vi "map_trap_switch_laser.vi"() -> ()   [LabVIEW 2015]
panel:
  out "Mapping file":string
  in  "Done ?":bool
  in  "KILL":bool
  in  "PAUSE":bool
  in  "RESUME":bool
  in  "QUIT":bool
  in  "up done":bool
  in  "z up":bool
  in  "Done":bool
  in  "z piastra":bool
  in  "y piastra":bool
  in  "x piastra":bool
  in  "goto x pos":bool
  in  "Panello o piastre?":bool
  in  "End":bool
  in  "zero z - end":bool
  in  "zero x - end":bool
  in  "zero y - end":bool
  in  "goto z pos":bool
  in  "positioning done":bool
  out "output":string
  out "command":string
  in  "zero done":bool
  in  "zero z":bool
  in  "zero x":bool
  in  "zero y":bool
  # "Comandi di emergenza"
  # "Mappatura a trapezio \nper il pannello e le piastre"
  # "In alto: TRUE ---> Panello"
  # "In basso: FALSE ---> Piastre"
  # "Posiziono in zero"
  # "Vado sulla piastra \ne azzero"
  # "Alzo il laser"
  # "Vado in posizione"
  # "Ritorno a zero"
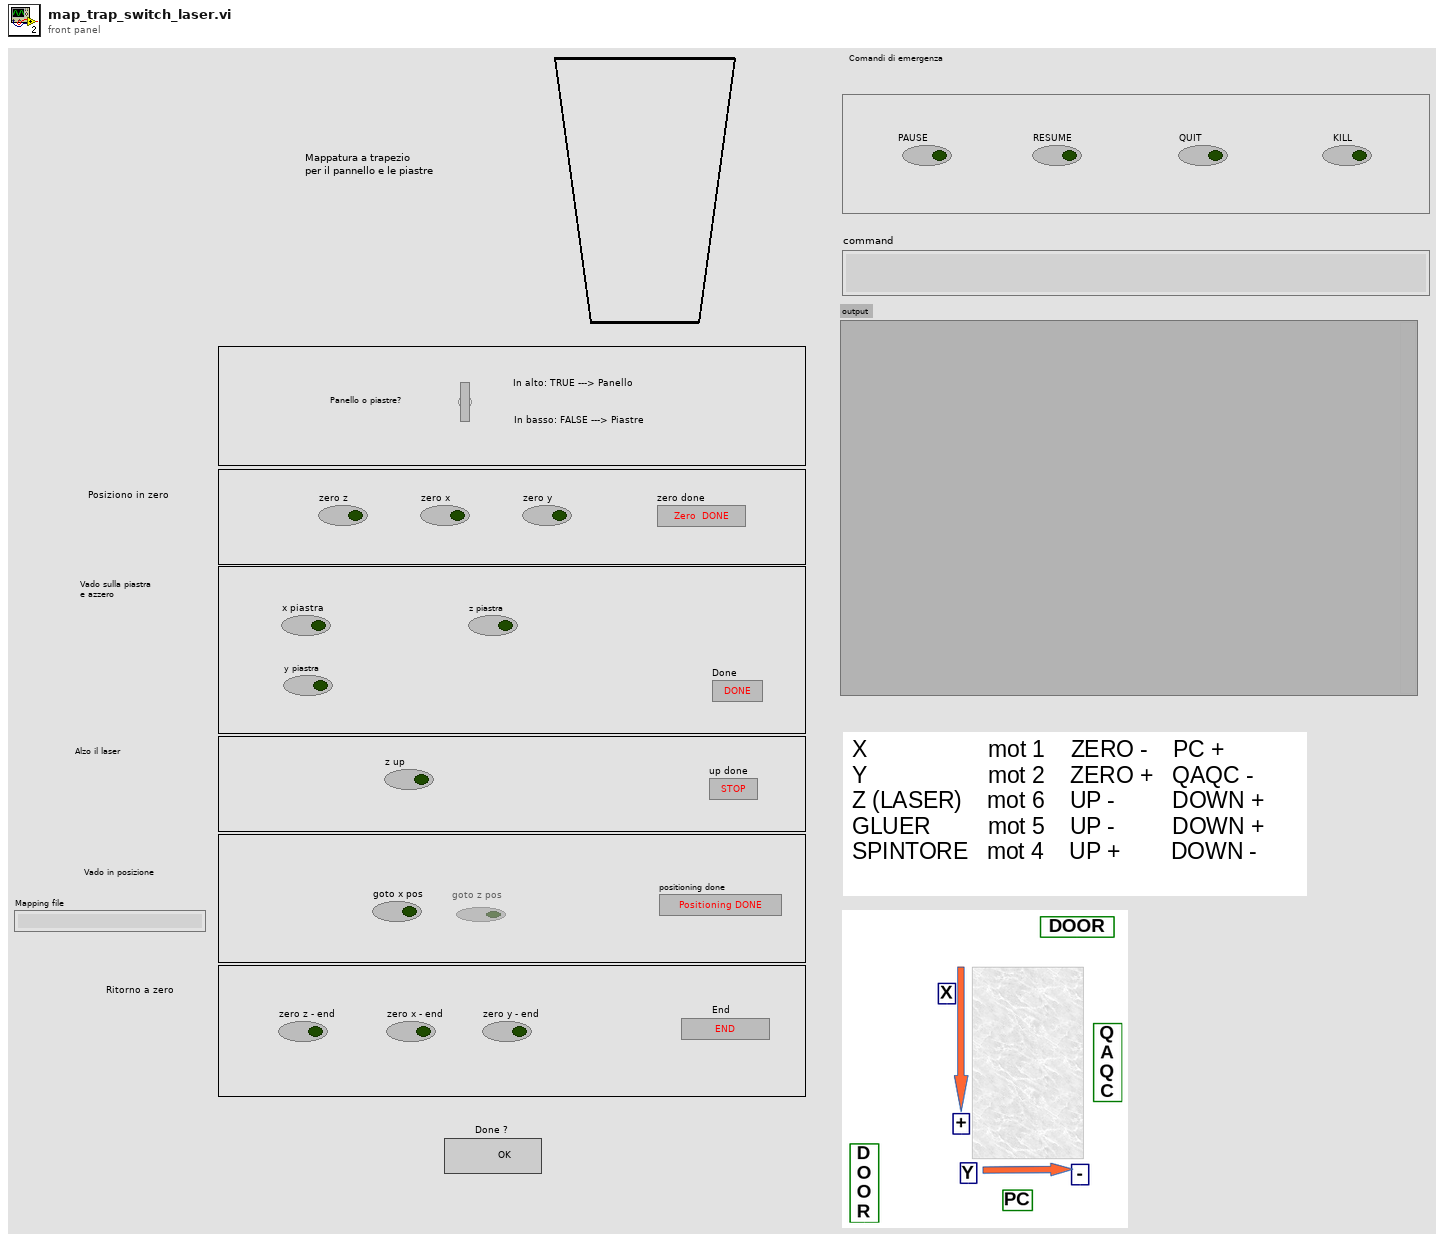
[diagram p1: front panel]
types:
  T1 = enum8{"Enabled", "Disabled", "Disabled and Grayed Out"}
  T2 = enum16{"open", "replace", "create", "open or create", "replace or create", "replace or create with confirmation"}
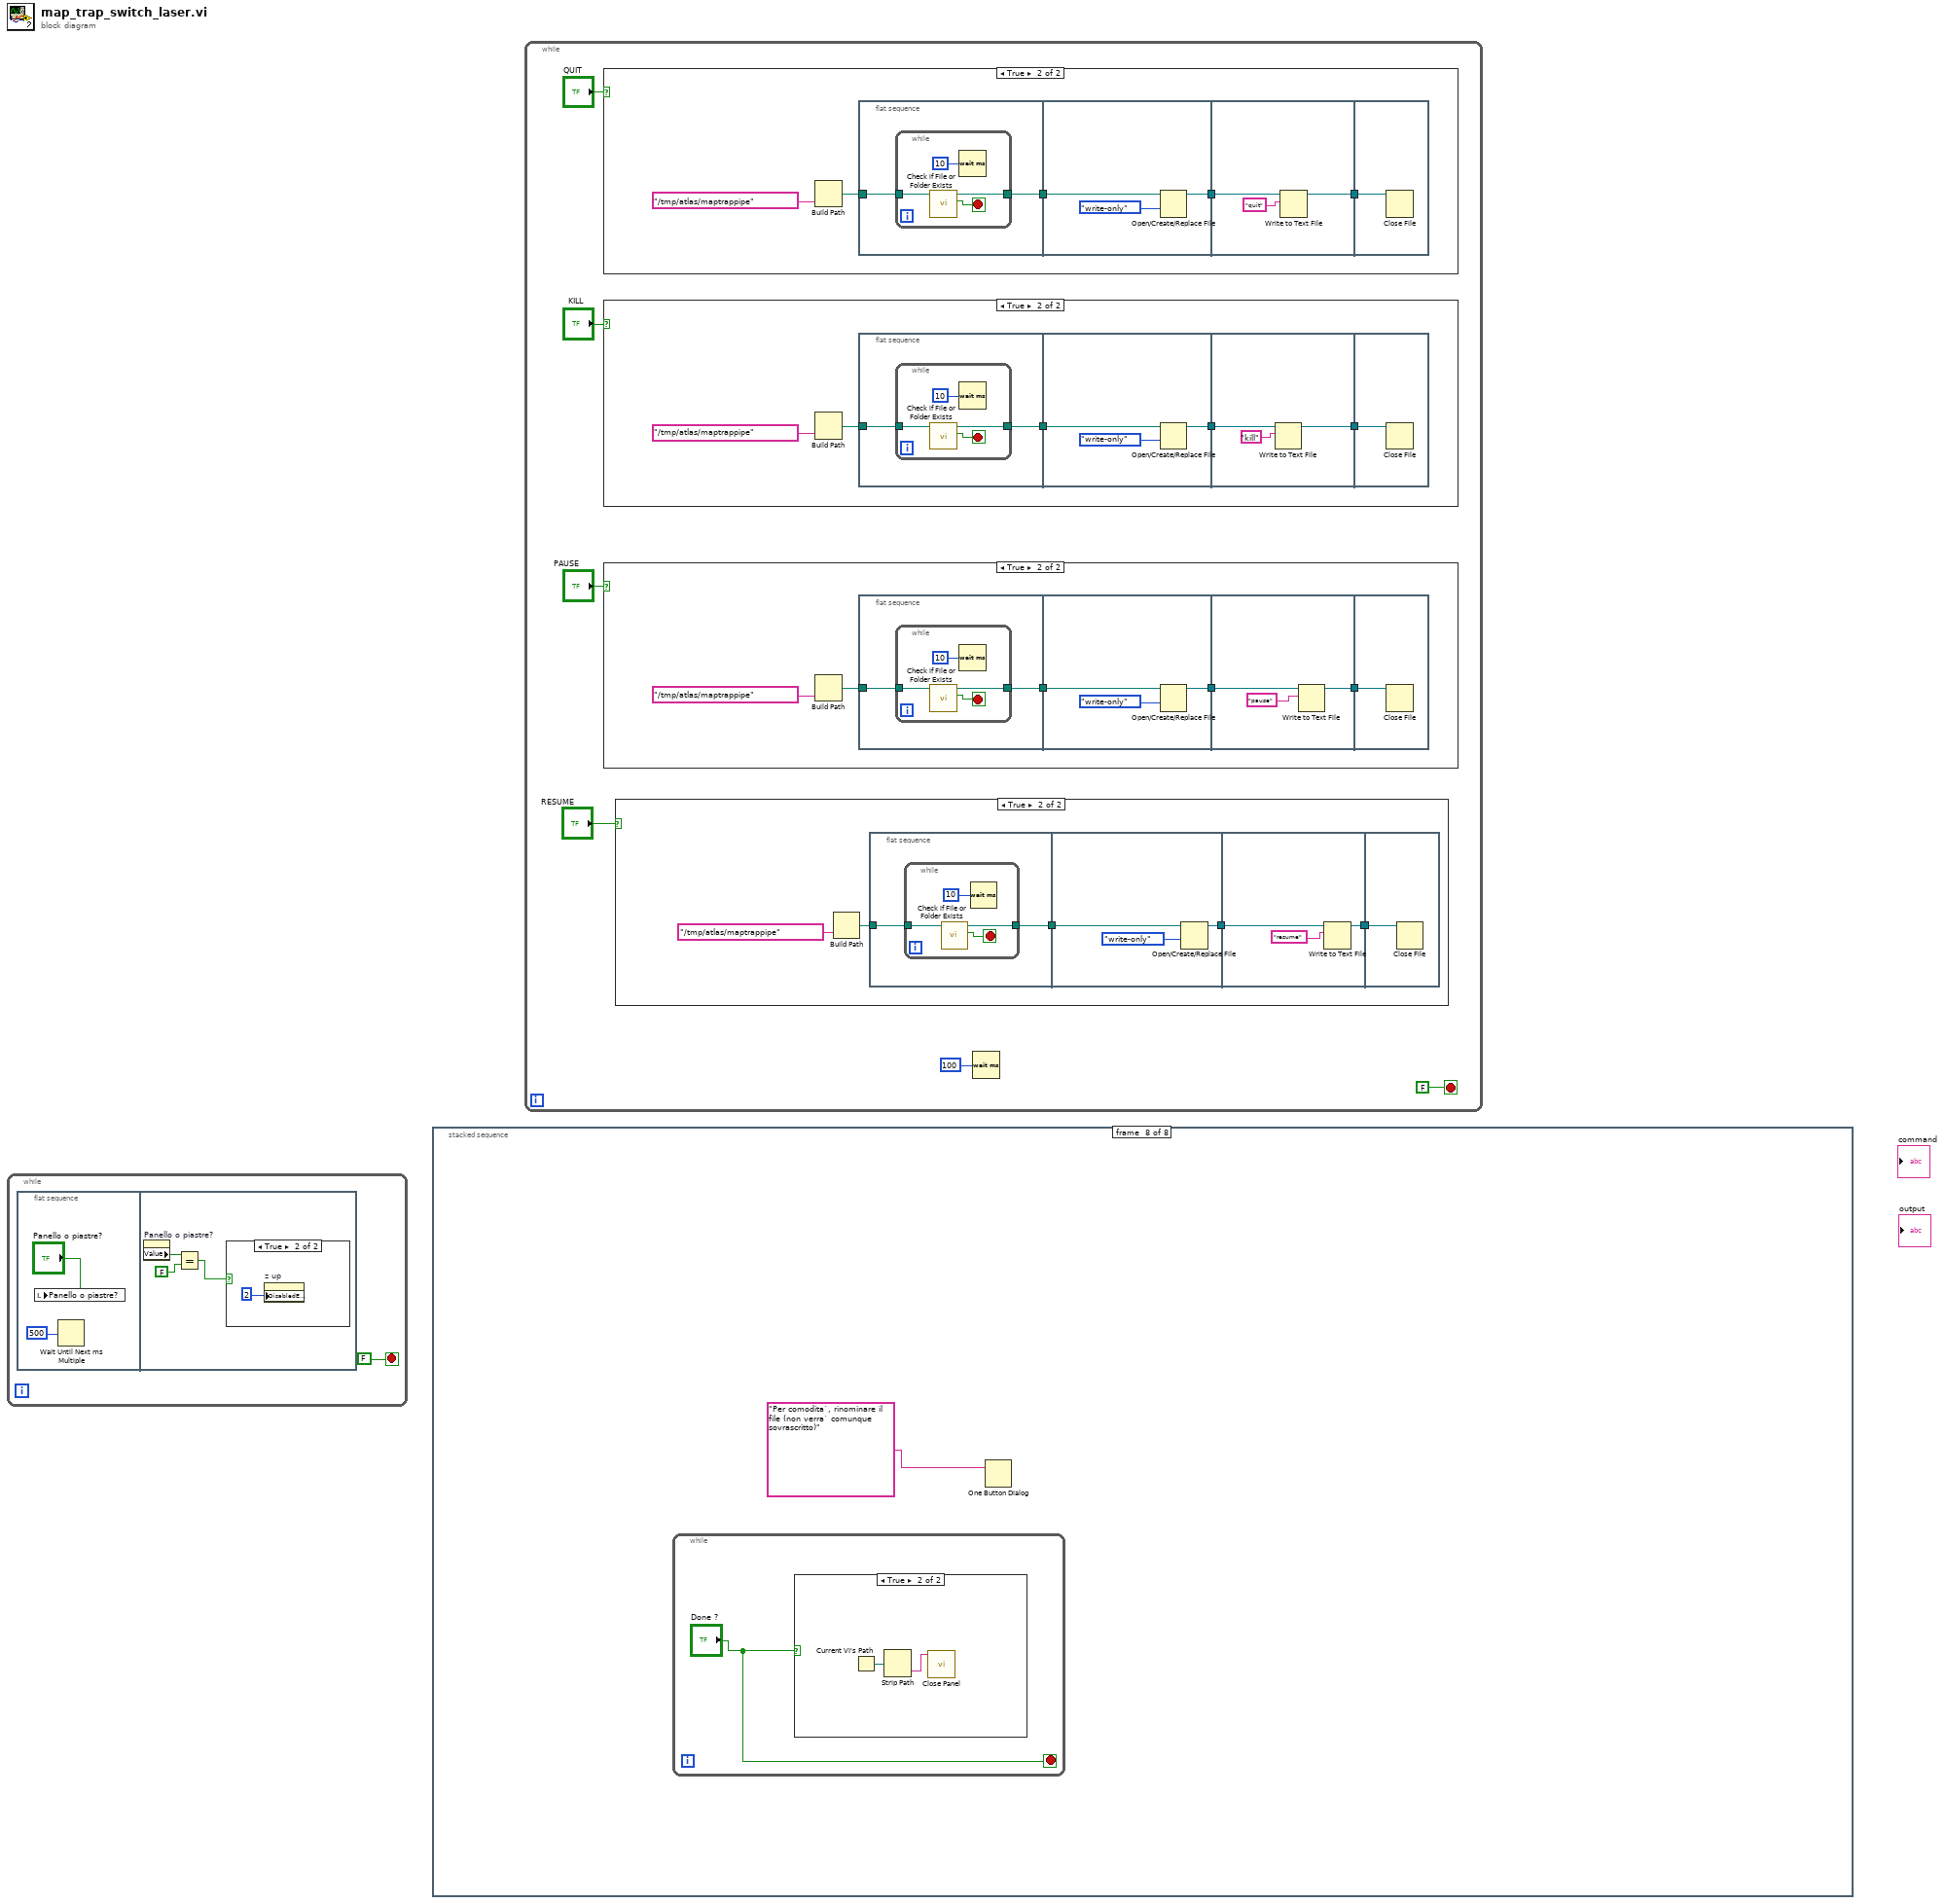
[diagram p0: block diagram]
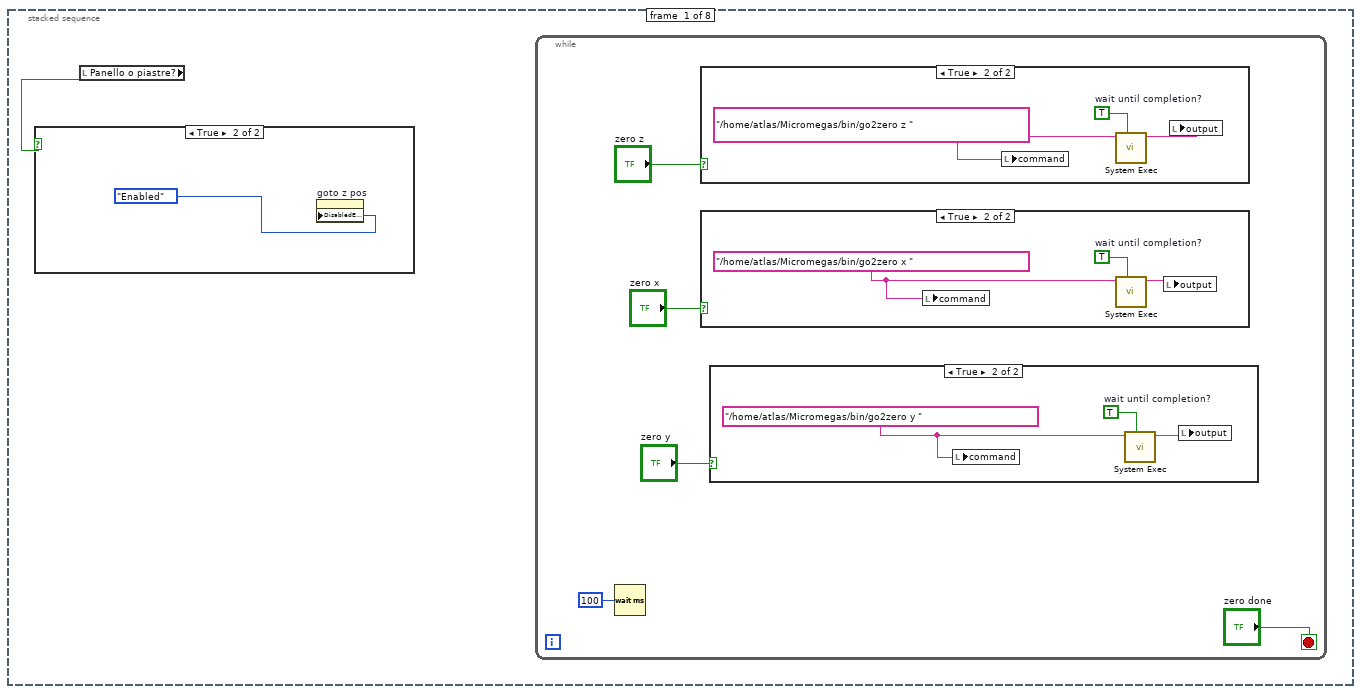
[diagram p7: hidden frame]
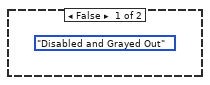
[diagram p8: hidden frame]
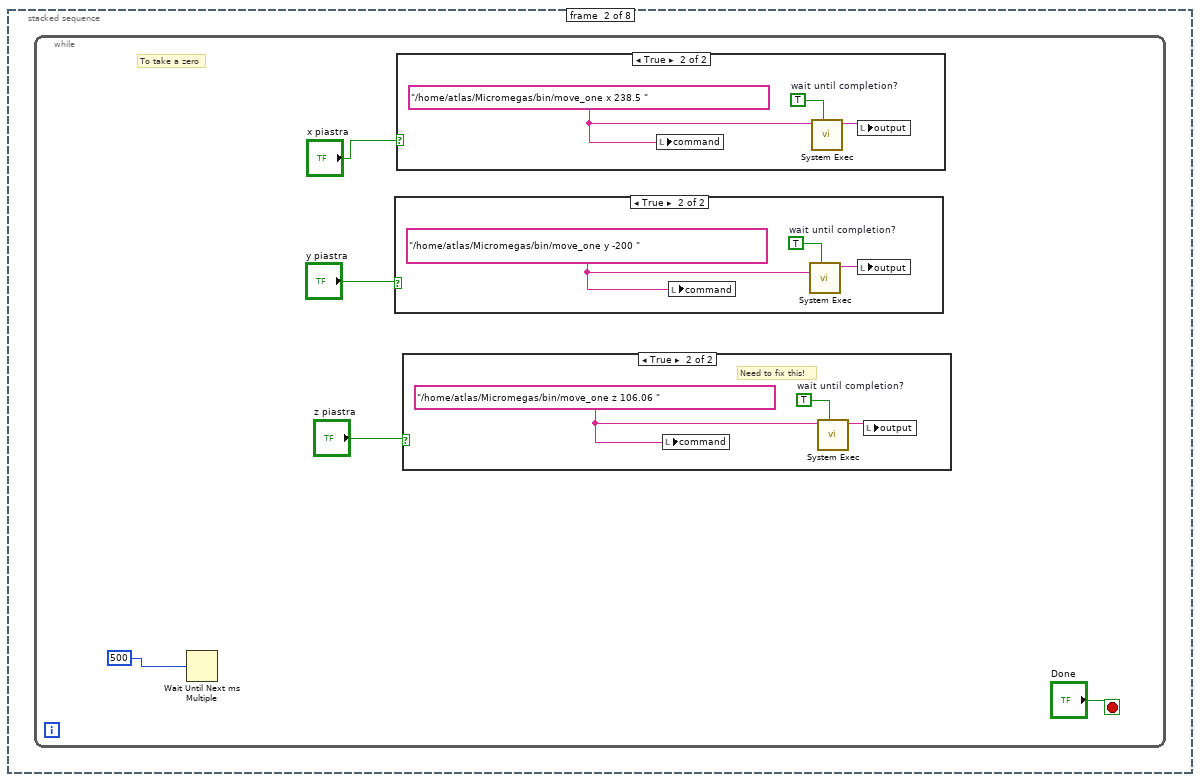
[diagram p12: hidden frame]
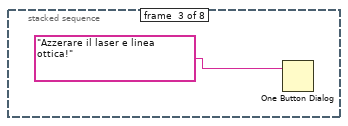
[diagram p16: hidden frame]
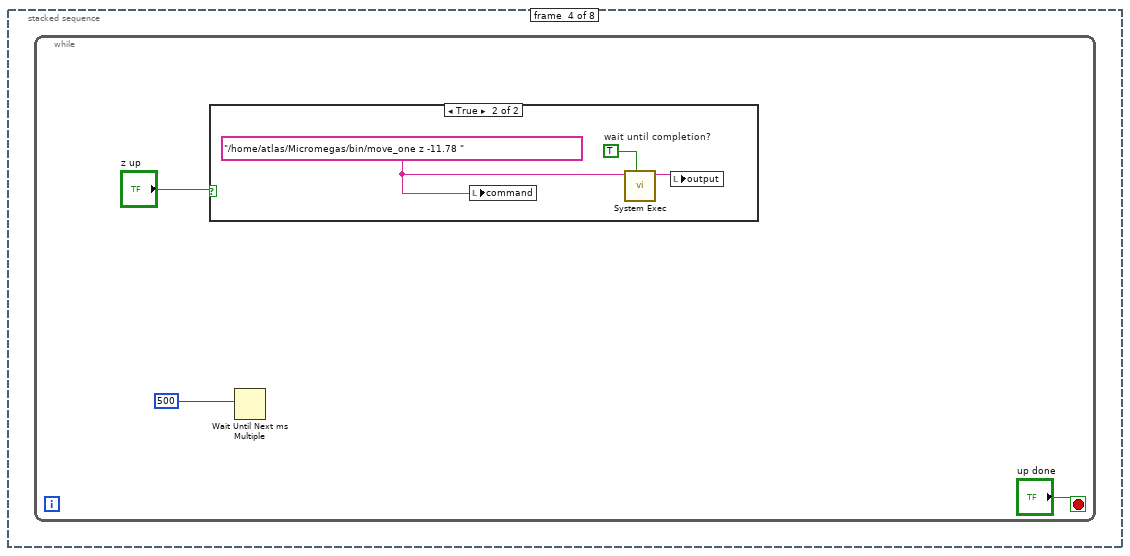
[diagram p17: hidden frame]
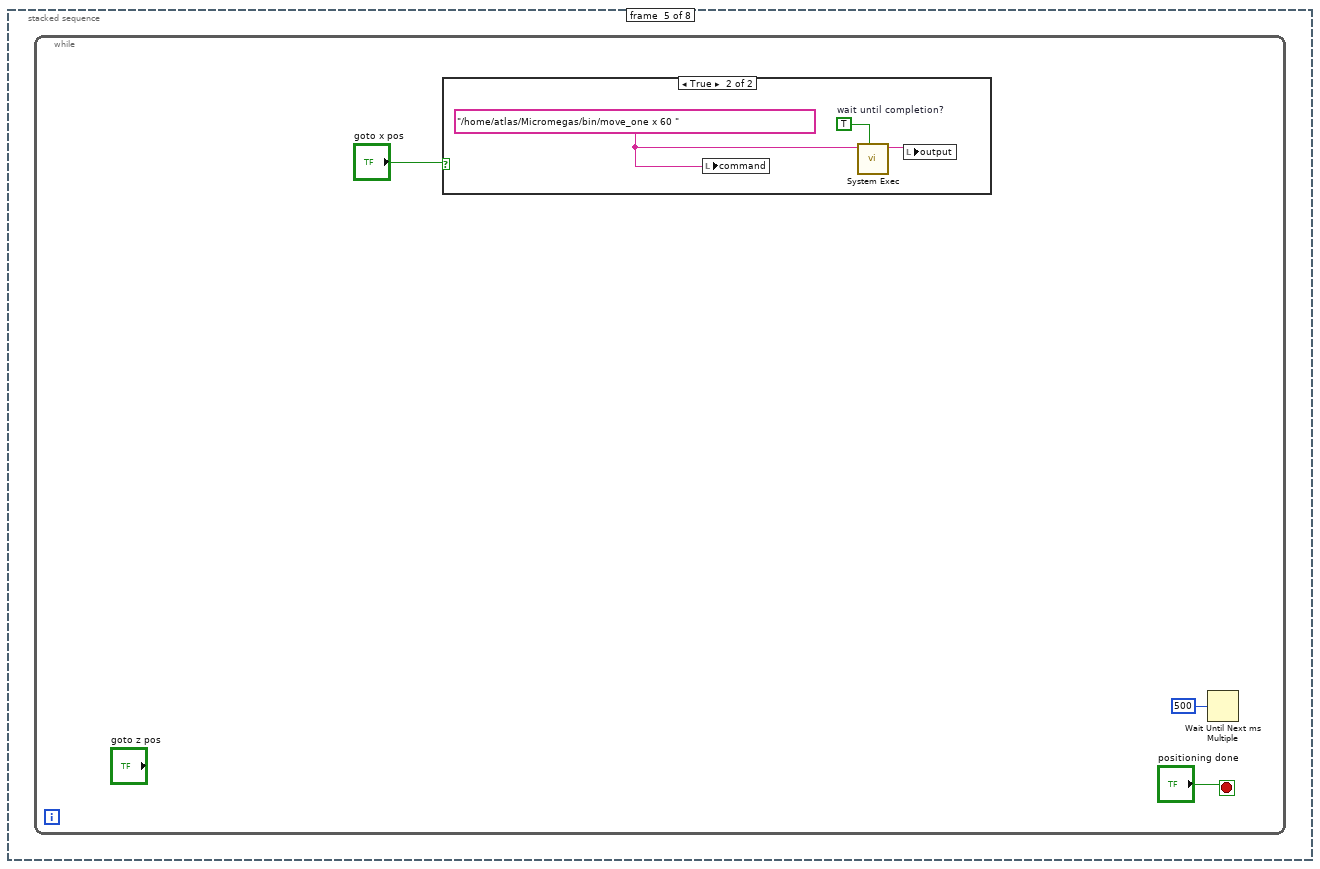
[diagram p19: hidden frame]
diagram:
  n1 = while {
    stop <- FALSE stop-if-true
    n2 = flat-sequence {
      frame #0 {
        n3 = local write "Panello o piastre?"("Panello o piastre?") -> ()
        n4 = Wait Until Next ms Multiple(millisecond multiple=u32 500) -> ()  [unwired: 1 out]
      }
      frame #1 {
        n5 = property on="Panello o piastre?" class="Bool (strict)"() -> ("Value"=w6:bool)  [unwired: 2 in, 2 out]
        n6 = Equal?(x=w6, y=FALSE) -> (x = y?=w4:bool)
        n7 = case shown="True" w4 {
          frame False {
          }
          frame True {
            n8 = property on="z up" class="Bool"("DisabledEnum"=2) -> ()  [unwired: 2 in, 2 out]
          }
        }
      }
    }
  }
  n9 = stacked-sequence {
    frame #0 {
      n10 = local read "Panello o piastre?"() -> (w8:bool)
      n11 = case shown="True" w8 {
        frame False {
          (unwired) T1."Disabled and Grayed Out" ("Disabled")
        }
        frame True {
          n12 = property on="goto z pos" class="Bool (strict)"("DisabledEnum"=T1."Enabled" ("Disabled")) -> ()  [unwired: 2 in, 2 out]
        }
      }
      n13 = while {
        stop <- "zero done" stop-if-true
        n14 = Wait (ms)(milliseconds to wait=u32 100) -> ()  [unwired: 1 out]
        n15 = case shown="True" "zero z" {
          frame False {
          }
          frame True {
            w22 = "/home/atlas/Micromegas/bin/go2zero z " ("string")
            w23 = TRUE  # wait until completion?
            n16 = local write "command"(w22) -> ()
            n17 = call <vilib>:"System Exec.vi"("wait until completion? (T)"=w23, "command line"=w22) -> ("standard output"=w21:string)  [unwired: 6 in, 3 out]
            n18 = local write "output"(w21) -> ()
          }
        }
        n19 = case shown="True" "zero x" {
          frame False {
          }
          frame True {
            w19 = "/home/atlas/Micromegas/bin/go2zero x " ("string")
            w20 = TRUE  # wait until completion?
            n20 = local write "command"(w19) -> ()
            n21 = call <vilib>:"System Exec.vi"("wait until completion? (T)"=w20, "command line"=w19) -> ("standard output"=w18:string)  [unwired: 6 in, 3 out]
            n22 = local write "output"(w18) -> ()
          }
        }
        n23 = case shown="True" "zero y" {
          frame False {
          }
          frame True {
            w16 = "/home/atlas/Micromegas/bin/go2zero y " ("string")
            w17 = TRUE  # wait until completion?
            n24 = local write "command"(w16) -> ()
            n25 = call <vilib>:"System Exec.vi"("wait until completion? (T)"=w17, "command line"=w16) -> ("standard output"=w15:string)  [unwired: 6 in, 3 out]
            n26 = local write "output"(w15) -> ()
          }
        }
      }
    }
    frame #1 {
      n27 = while {
        stop <- "Done" stop-if-true
        # "To take a zero"
        n28 = Wait Until Next ms Multiple(millisecond multiple=u32 500 ("millisecond timer value")) -> ()  [unwired: 1 out]
        n29 = case shown="True" "y piastra" {
          frame False {
          }
          frame True {
            w32 = "/home/atlas/Micromegas/bin/move_one y -200 " ("string")
            w34 = TRUE  # wait until completion?
            n30 = local write "command"(w32) -> ()
            n31 = call <vilib>:"System Exec.vi"("wait until completion? (T)"=w34, "command line"=w32) -> ("standard output"=w33:string)  [unwired: 6 in, 3 out]
            n32 = local write "output"(w33) -> ()
          }
        }
        n33 = case shown="True" "x piastra" {
          frame False {
          }
          frame True {
            w35 = "/home/atlas/Micromegas/bin/move_one x 238.5 " ("string")
            w37 = TRUE  # wait until completion?
            n34 = local write "command"(w35) -> ()
            n35 = call <vilib>:"System Exec.vi"("wait until completion? (T)"=w37, "command line"=w35) -> ("standard output"=w36:string)  [unwired: 6 in, 3 out]
            n36 = local write "output"(w36) -> ()
          }
        }
        n37 = case shown="True" "z piastra" {
          frame False {
          }
          frame True {
            w29 = "/home/atlas/Micromegas/bin/move_one z 106.06 " ("string")
            w31 = TRUE  # wait until completion?
            # "Need to fix this!"
            n38 = local write "command"(w29) -> ()
            n39 = call <vilib>:"System Exec.vi"("wait until completion? (T)"=w31, "command line"=w29) -> ("standard output"=w30:string)  [unwired: 6 in, 3 out]
            n40 = local write "output"(w30) -> ()
          }
        }
      }
    }
    frame #2 {
      n41 = One Button Dialog(message="Azzerare il laser e linea ottica!") -> ()  [unwired: 1 in, 1 out]
    }
    frame #3 {
      n42 = while {
        stop <- "up done" stop-if-true
        n43 = case shown="True" "z up" {
          frame False {
          }
          frame True {
            w42 = "/home/atlas/Micromegas/bin/move_one z -11.78 " ("string")
            w44 = TRUE  # wait until completion?
            n44 = local write "command"(w42) -> ()
            n45 = call <vilib>:"System Exec.vi"("wait until completion? (T)"=w44, "command line"=w42) -> ("standard output"=w43:string)  [unwired: 6 in, 3 out]
            n46 = local write "output"(w43) -> ()
          }
        }
        n47 = Wait Until Next ms Multiple(millisecond multiple=u32 500 ("millisecond timer value")) -> ()  [unwired: 1 out]
      }
    }
    frame #4 {
      n48 = while {
        stop <- "positioning done" stop-if-true
        n49 = case shown="True" "goto x pos" {
          frame False {
          }
          frame True {
            w48 = "/home/atlas/Micromegas/bin/move_one x 60 " ("string")
            w50 = TRUE  # wait until completion?
            n50 = local write "command"(w48) -> ()
            n51 = call <vilib>:"System Exec.vi"("wait until completion? (T)"=w50, "command line"=w48) -> ("standard output"=w49:string)  [unwired: 6 in, 3 out]
            n52 = local write "output"(w49) -> ()
          }
        }
        n53 = Wait Until Next ms Multiple(millisecond multiple=u32 500) -> ()  [unwired: 1 out]
      }
    }
    frame #5 {
      n54 = flat-sequence {
        frame #0 {
          # "Show the last lines continiously"
          n55 = Open/Create/Replace File(file path (use dialog)=path "/tmp/map_trap.tmp", operation (0:open)=T2."open or create") -> ()  [unwired: 4 in, 3 out]
          n56 = call <vilib>:"System Exec.vi"("wait until completion? (T)"=FALSE, "command line"="gnome-terminal -e \"tail -f /tmp/map_trap.tmp\"") -> ()  [unwired: 6 in, 4 out]
        }
        frame #1 {
          w61 = TRUE  # wait until completion?
          # "Write the tail output to a temp file"
          # "Runs the map_trap executable with some arguments"
          # "W: x length, y length\nX: x step, x speed\nY: y step, y speed\nT: z step, z speed"
          n57 = Concatenate Strings("/home/atlas/Micromegas/bin/map_trap_laser_step  " ("string"), "" ("string"), "-w 2070 1001 -x 90 20 -y 77 20" ("string"), "  | tee /tmp/map_trap.tmp" ("string")) -> (w56:string)
          n58 = local write "command"(w56) -> ()
          n59 = call <vilib>:"System Exec.vi"("wait until completion? (T)"=w61, "command line"=w56) -> ("standard output"=w55:string)  [unwired: 6 in, 3 out]
          n60 = local write "output"(w55) -> ()
        }
        frame #2 {
          n61 = Open/Create/Replace File(file path (use dialog)=path "/M05Data/mapping/map_trap_filename.txt", operation (0:open)=T2."open") -> (refnum out=w64:refnum<file>, error out=w63:errorcluster)  [unwired: 4 in, 1 out]
          n62 = Read from Text File(file (use dialog)=w64, error in=w63) -> (text=→"Mapping file":string)  [unwired: 2 in, 3 out]
        }
      }
    }
    frame #6 {
      n63 = while {
        stop <- "End" stop-if-true
        n64 = Wait (ms)(milliseconds to wait=u32 100) -> ()  [unwired: 1 out]
        n65 = case shown="True" "zero z - end" {
          frame False {
          }
          frame True {
            w79 = "/home/atlas/Micromegas/bin/go2zero z " ("string")
            w80 = TRUE  # wait until completion?
            n66 = local write "command"(w79) -> ()
            n67 = call <vilib>:"System Exec.vi"("wait until completion? (T)"=w80, "command line"=w79) -> ("standard output"=w78:string)  [unwired: 6 in, 3 out]
            n68 = local write "output"(w78) -> ()
          }
        }
        n69 = case shown="True" "zero x - end" {
          frame False {
          }
          frame True {
            w76 = "/home/atlas/Micromegas/bin/go2zero x " ("string")
            w77 = TRUE  # wait until completion?
            n70 = local write "command"(w76) -> ()
            n71 = call <vilib>:"System Exec.vi"("wait until completion? (T)"=w77, "command line"=w76) -> ("standard output"=w75:string)  [unwired: 6 in, 3 out]
            n72 = local write "output"(w75) -> ()
          }
        }
        n73 = case shown="True" "zero y - end" {
          frame False {
          }
          frame True {
            w73 = "/home/atlas/Micromegas/bin/go2zero y " ("string")
            w74 = TRUE  # wait until completion?
            n74 = local write "command"(w73) -> ()
            n75 = call <vilib>:"System Exec.vi"("wait until completion? (T)"=w74, "command line"=w73) -> ("standard output"=w72:string)  [unwired: 6 in, 3 out]
            n76 = local write "output"(w72) -> ()
          }
        }
      }
    }
    frame #7 {
      n77 = while {
        stop <- "Done ?" stop-if-true
        n78 = case shown="True" "Done ?" {
          frame False {
          }
          frame True {
            n79 = Current VI's Path() -> (path=w83:path)
            n80 = Strip Path(path=w83) -> (name=w84:string)  [unwired: 1 out]
            n81 = call <vilib>:"Close Panel.vi"("VI name"=w84) -> ()  [unwired: 10 in, 1 out]
          }
        }
      }
      n82 = One Button Dialog(message="Per comodita`, rinominare il file (non verra` comunque sovrascritto)") -> ()  [unwired: 1 in, 1 out]
    }
  }
  n83 = while {
    stop <- FALSE stop-if-true
    n84 = case shown="True" "QUIT" {
      frame False {
      }
      frame True {
        n85 = Build Path(name or relative path="/tmp/atlas/maptrappipe" ("string")) -> (appended path=w145:path)  [unwired: 1 in]
        n86 = flat-sequence {
          tunnel: [w151] -> w149
          tunnel: w145 -> [w150]
          tunnel: w149 -> [w158]
          tunnel: [w156] -> w148
          tunnel: w148 -> [w161]
          tunnel: [w160] -> w147
          tunnel: w147 -> [w162]
          frame #0 {
            n87 = while {
              tunnel: [w153] -> w151
              tunnel: w150 -> [w152]
              stop <- w154 stop-if-true
              n88 = call <vilib>:"Check if File or Folder Exists.vi"("path"=w152) -> ("file or folder exists?"=w154:bool, "dup path"=w153:path)  [unwired: 8 in, 1 out]
              n89 = Wait (ms)(milliseconds to wait=u32 10) -> ()  [unwired: 1 out]
            }
          }
          frame #1 {
            n90 = Open/Create/Replace File(file path (use dialog)=w158, access (0:read/write)=enum16{"read/write", "read-only", "write-only"}."write-only") -> (refnum out=w156:refnum<file>)  [unwired: 4 in, 2 out]
          }
          frame #2 {
            n91 = Write to Text File(file (use dialog)=w161, text="quit") -> (refnum out=w160:refnum<file>)  [unwired: 2 in, 2 out]
          }
          frame #3 {
            n92 = Close File(refnum=w162) -> ()  [unwired: 1 in, 2 out]
          }
        }
      }
    }
    n93 = case shown="True" "KILL" {
      frame False {
      }
      frame True {
        n94 = Build Path(name or relative path="/tmp/atlas/maptrappipe" ("string")) -> (appended path=w109:path)  [unwired: 1 in]
        n95 = flat-sequence {
          tunnel: [w115] -> w113
          tunnel: w109 -> [w114]
          tunnel: w113 -> [w122]
          tunnel: [w120] -> w112
          tunnel: w112 -> [w125]
          tunnel: [w124] -> w111
          tunnel: w111 -> [w126]
          frame #0 {
            n96 = while {
              tunnel: [w117] -> w115
              tunnel: w114 -> [w116]
              stop <- w118 stop-if-true
              n97 = call <vilib>:"Check if File or Folder Exists.vi"("path"=w116) -> ("file or folder exists?"=w118:bool, "dup path"=w117:path)  [unwired: 8 in, 1 out]
              n98 = Wait (ms)(milliseconds to wait=u32 10) -> ()  [unwired: 1 out]
            }
          }
          frame #1 {
            n99 = Open/Create/Replace File(file path (use dialog)=w122, access (0:read/write)=enum16{"read/write", "read-only", "write-only"}."write-only") -> (refnum out=w120:refnum<file>)  [unwired: 4 in, 2 out]
          }
          frame #2 {
            n100 = Write to Text File(file (use dialog)=w125, text="kill") -> (refnum out=w124:refnum<file>)  [unwired: 2 in, 2 out]
          }
          frame #3 {
            n101 = Close File(refnum=w126) -> ()  [unwired: 1 in, 2 out]
          }
        }
      }
    }
    n102 = case shown="True" "PAUSE" {
      frame False {
      }
      frame True {
        n103 = Build Path(name or relative path="/tmp/atlas/maptrappipe" ("string")) -> (appended path=w91:path)  [unwired: 1 in]
        n104 = flat-sequence {
          tunnel: [w97] -> w95
          tunnel: w91 -> [w96]
          tunnel: w95 -> [w104]
          tunnel: [w102] -> w94
          tunnel: w94 -> [w107]
          tunnel: [w106] -> w93
          tunnel: w93 -> [w108]
          frame #0 {
            n105 = while {
              tunnel: [w99] -> w97
              tunnel: w96 -> [w98]
              stop <- w100 stop-if-true
              n106 = call <vilib>:"Check if File or Folder Exists.vi"("path"=w98) -> ("file or folder exists?"=w100:bool, "dup path"=w99:path)  [unwired: 8 in, 1 out]
              n107 = Wait (ms)(milliseconds to wait=u32 10) -> ()  [unwired: 1 out]
            }
          }
          frame #1 {
            n108 = Open/Create/Replace File(file path (use dialog)=w104, access (0:read/write)=enum16{"read/write", "read-only", "write-only"}."write-only") -> (refnum out=w102:refnum<file>)  [unwired: 4 in, 2 out]
          }
          frame #2 {
            n109 = Write to Text File(file (use dialog)=w107, text="pause") -> (refnum out=w106:refnum<file>)  [unwired: 2 in, 2 out]
          }
          frame #3 {
            n110 = Close File(refnum=w108) -> ()  [unwired: 1 in, 2 out]
          }
        }
      }
    }
    n111 = case shown="True" "RESUME" {
      frame False {
      }
      frame True {
        n112 = Build Path(name or relative path="/tmp/atlas/maptrappipe" ("string")) -> (appended path=w127:path)  [unwired: 1 in]
        n113 = flat-sequence {
          tunnel: [w133] -> w131
          tunnel: w127 -> [w132]
          tunnel: w131 -> [w140]
          tunnel: [w138] -> w130
          tunnel: w130 -> [w143]
          tunnel: [w142] -> w129
          tunnel: w129 -> [w144]
          frame #0 {
            n114 = while {
              tunnel: [w135] -> w133
              tunnel: w132 -> [w134]
              stop <- w136 stop-if-true
              n115 = call <vilib>:"Check if File or Folder Exists.vi"("path"=w134) -> ("file or folder exists?"=w136:bool, "dup path"=w135:path)  [unwired: 8 in, 1 out]
              n116 = Wait (ms)(milliseconds to wait=u32 10) -> ()  [unwired: 1 out]
            }
          }
          frame #1 {
            n117 = Open/Create/Replace File(file path (use dialog)=w140, access (0:read/write)=enum16{"read/write", "read-only", "write-only"}."write-only") -> (refnum out=w138:refnum<file>)  [unwired: 4 in, 2 out]
          }
          frame #2 {
            n118 = Write to Text File(file (use dialog)=w143, text="resume") -> (refnum out=w142:refnum<file>)  [unwired: 2 in, 2 out]
          }
          frame #3 {
            n119 = Close File(refnum=w144) -> ()  [unwired: 1 in, 2 out]
          }
        }
      }
    }
    n120 = Wait (ms)(milliseconds to wait=100) -> ()  [unwired: 1 out]
  }
